vi "Dac_release_all_lines.vi"(11 "Release all DAQ lines":bool) -> (3 "Finished":bool)   [LabVIEW 2020]
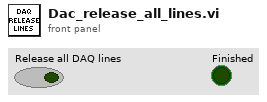
[diagram p1: front panel]
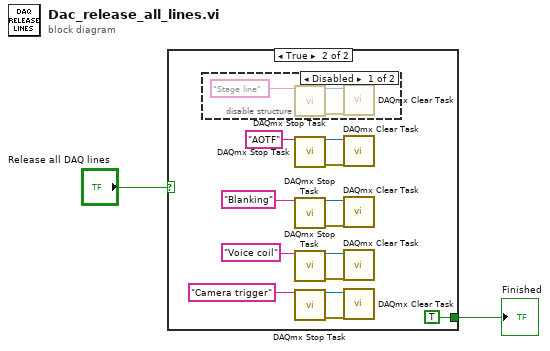
[diagram p0: block diagram]
diagram:
  n1 = case shown="True" "Release all DAQ lines" {
    tunnel: [_ TRUE] -> w1
    frame False {
    }
    frame True {
      n2 = disable-structure shown="Disabled" {
        frame Disabled {
          n3 = call <vilib>:"DAQmx Stop Task.vi"("task/channels in"="Stage line") -> ("task out"=w18:refnum<k21>, "error out"=w17:errorcluster)  [unwired: 13 in]
          n4 = call <vilib>:"DAQmx Clear Task.vi"("task in"=w18, "error in"=w17) -> ()  [unwired: 13 in, 1 out]
        }
        frame Enabled {
        }
      }
      n5 = call <vilib>:"DAQmx Stop Task.vi"("task/channels in"="AOTF") -> ("task out"=w15:refnum<k21>, "error out"=w14:errorcluster)  [unwired: 13 in]
      n6 = call <vilib>:"DAQmx Stop Task.vi"("task/channels in"="Blanking") -> ("task out"=w11:refnum<k21>, "error out"=w10:errorcluster)  [unwired: 13 in]
      n7 = call <vilib>:"DAQmx Stop Task.vi"("task/channels in"="Voice coil") -> ("task out"=w8:refnum<k21>, "error out"=w7:errorcluster)  [unwired: 13 in]
      n8 = call <vilib>:"DAQmx Stop Task.vi"("task/channels in"="Camera trigger") -> ("task out"=w5:refnum<k21>, "error out"=w4:errorcluster)  [unwired: 13 in]
      n9 = call <vilib>:"DAQmx Clear Task.vi"("task in"=w15, "error in"=w14) -> ()  [unwired: 13 in, 1 out]
      n10 = call <vilib>:"DAQmx Clear Task.vi"("task in"=w11, "error in"=w10) -> ()  [unwired: 13 in, 1 out]
      n11 = call <vilib>:"DAQmx Clear Task.vi"("task in"=w8, "error in"=w7) -> ()  [unwired: 13 in, 1 out]
      n12 = call <vilib>:"DAQmx Clear Task.vi"("task in"=w5, "error in"=w4) -> ()  [unwired: 13 in, 1 out]
    }
  }
  "Finished" <- w1
